vi "Agilent_ScanList_Permutation.vi"(9 "Input Data Array":dbl[](array[numeric]), 10 "Agilent Scan List":string="111,112,113,114,115,116,109,110,313,201,202,203,204,205,206,207,208,209,210,211,212,213,214,215,216,107,108,314,315,316,105,106,301,302,303,304,305,306,307,308,309,310,311,312,101,102,103,104") -> (1 "Output Data Permutation":dbl[](array[numeric]))   [LabVIEW 2012]
panel:
  out "sorted array":i32[](array[numeric])
  out "number":i32[](array[numeric])
  out "Array":string[](array[string])
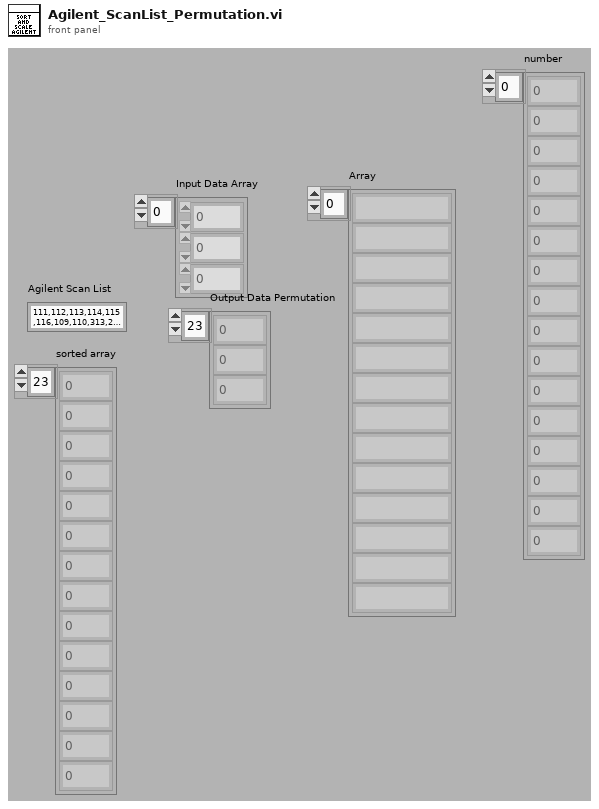
[diagram p1: front panel]
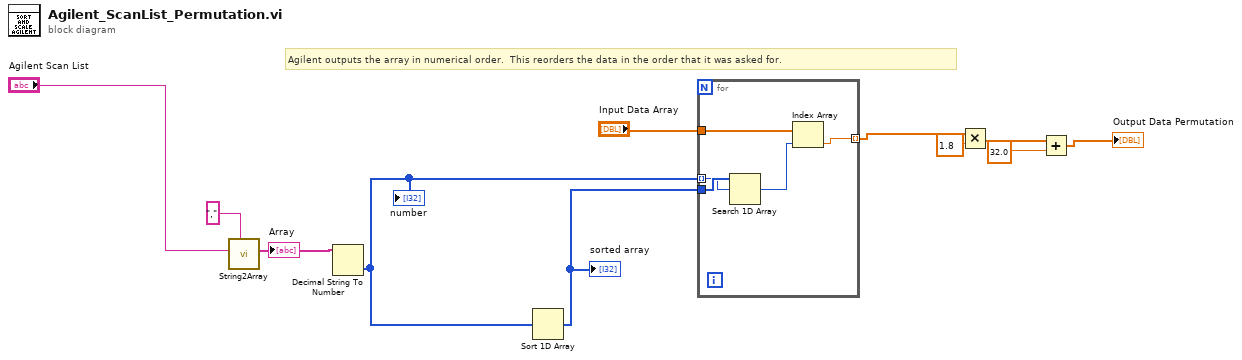
[diagram p0: block diagram]
diagram:
  # "Agilent outputs the array in numerical order.  This reorders the data in the order that it was asked for."
  n1 = call "String2Array.vi"("Delimiter"=",", "String"="Agilent Scan List") -> ("Array"=w8:string[])  [unwired: 9 in]
  "Array" <- w8
  n2 = Decimal String To Number(string=w8) -> (number=w6:i32[])  [unwired: 2 in, 1 out]
  "number" <- w6
  n3 = Sort 1D Array(array=w6) -> (sorted array=w7:i32[])
  "sorted array" <- w7
  n4 = for {
    tunnel: "Input Data Array" -> [w16]
    tunnel: [w15] -> w2 mode=indexing
    tunnel: w7 -> [w13]
    tunnel: w6 -> [w12] mode=indexing
    n5 = Search 1D Array(1D array=w13, element=w12) -> (index of element=w14:i32)  [unwired: 1 in]
    n6 = Index Array(array=w16, index=w14) -> (element=w15:dbl)
  }
  n7 = Multiply(x=w2, y=1.8) -> (x*y=w4:dbl[])
  n8 = Add(x=w4, y=32.0) -> (x+y=→"Output Data Permutation":dbl[])
